vi "RichToFlatnixnet_grpc_DbAddAliasRequest.vi"(5 "OutputClusterType":T1, 11 "InputCluster":T2) -> (3 "OutputCluster":T1)   [LabVIEW 2025, in "grpc-xnet_client.lvlib"]
uses:
  grpc-xnet_client.lvlib
  nixnet_grpc_DbAddAliasRequest.ctl
  nixnet_grpc_DbAddAliasRequest_Flat.ctl
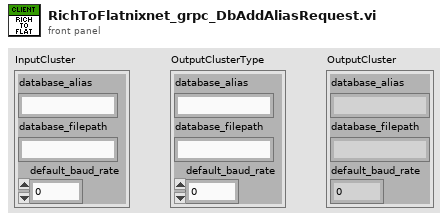
[diagram p1: front panel]
types:
  T1 = typedef "grpc-xnet_client.lvlib/nixnet_grpc_DbAddAliasRequest_Flat.ctl" = cluster{"database_alias":string, "database_filepath":string, "default_baud_rate":u32}
  T2 = typedef "grpc-xnet_client.lvlib/nixnet_grpc_DbAddAliasRequest.ctl" = cluster{"database_alias":string, "database_filepath":string, "default_baud_rate":u32}
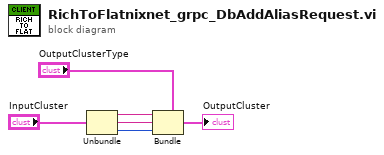
[diagram p0: block diagram]
diagram:
  n1 = Unbundle "Unbundle"("InputCluster") -> ("database_alias"=w3:string, "database_filepath"=w2:string, "default_baud_rate"=w1:u32)
  n2 = Bundle "Bundle"(cluster="OutputClusterType", "database_alias"=w3, "database_filepath"=w2, "default_baud_rate"=w1) -> (→"OutputCluster":T1)
